vi "DumbDash Load Values.vi"(7 "Message Box":refnum<vi>, 10 "Robot":T1, 11 "Controls In":T2[](array[typedef])) -> ()   [LabVIEW 2017]
uses:
  DumbDash Control.ctl
  DumbDash Control Type.ctl
  Common Code/Robot Name.ctl
  <vilib>/Utility/sysdir.llb/System Directory Type.ctl
  <vilib>/Utility/config.llb/Read Key (Double).vi
  <vilib>/Utility/config.llb/Read Key (Boolean).vi
  <vilib>/Utility/config.llb/Read Key (String).vi
  <vilib>/Utility/config.llb/NI_LVConfig.lvlib
panel:
  out "file path":path
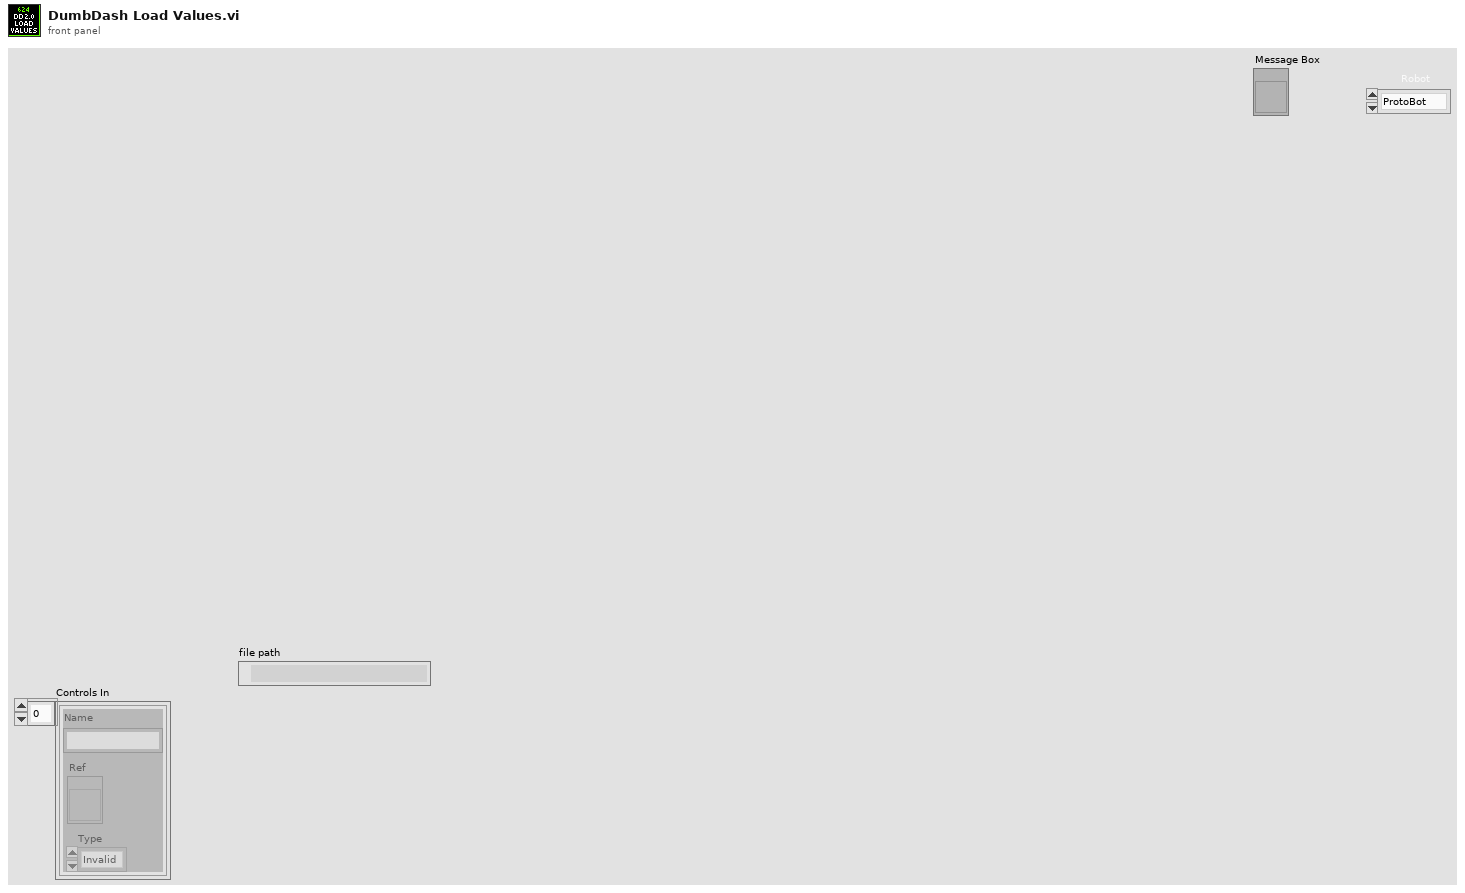
[diagram p1: front panel]
types:
  T1 = typedef "Robot Name.ctl" = enum16{"ProtoBot", "Main Robot", "Practice Robot"}
  T2 = typedef "DumbDash Control.ctl" = cluster{"Name":string, "Ref":refnum<vi>, "Type":T3}
  T3 = typedef "DumbDash Control Type.ctl" = enum16{"Invalid", "Number", "Boolean", "String"}
  T4 = typedef "System Directory Type.ctl" = i32
  T5 = typedef "NI_LVConfig.lvlib/Config Data RefNum.ctl" = refnum<k1>
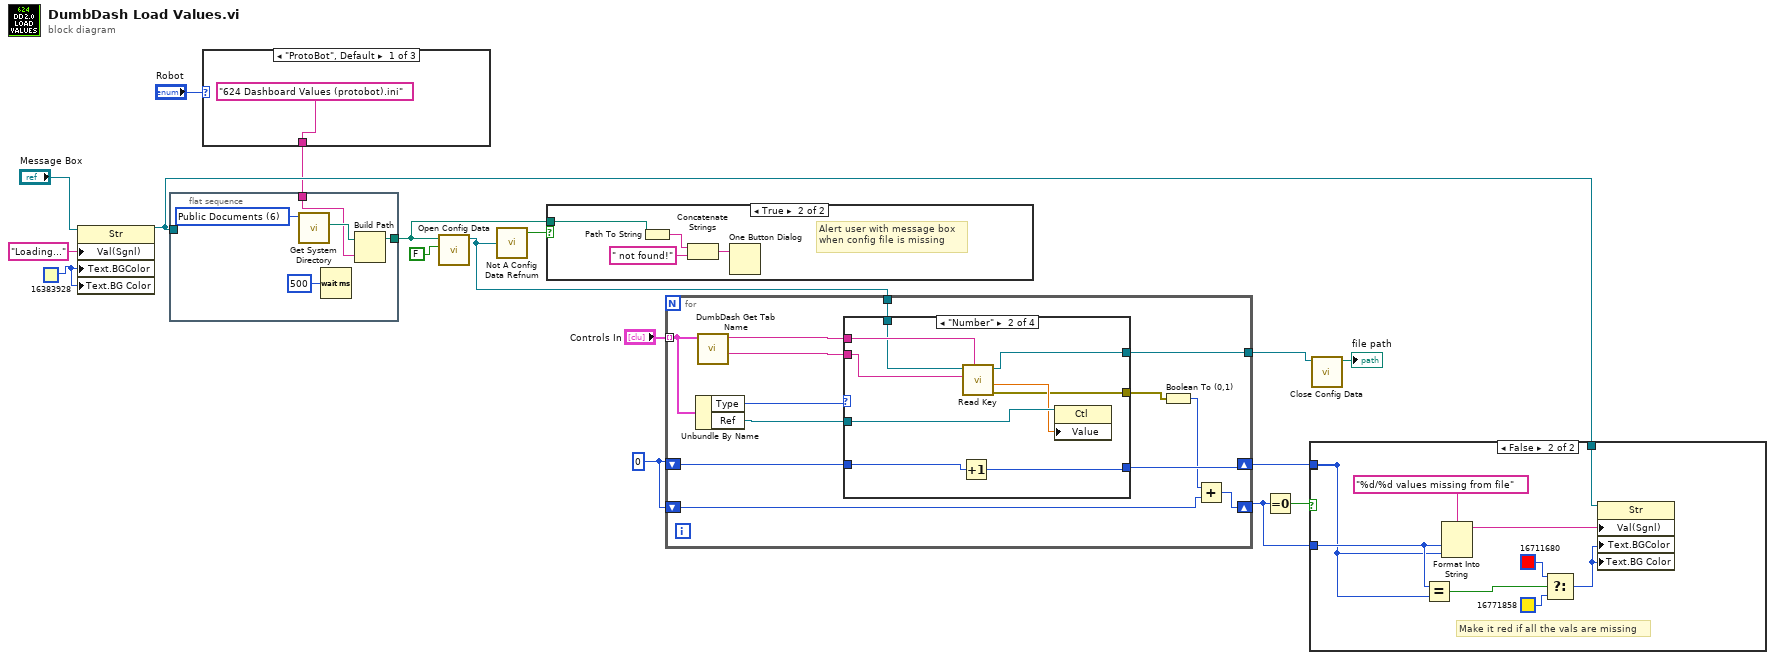
[diagram p0: block diagram]
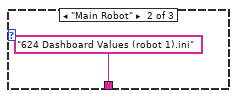
[diagram p2: hidden frame]
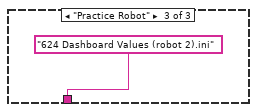
[diagram p3: hidden frame]
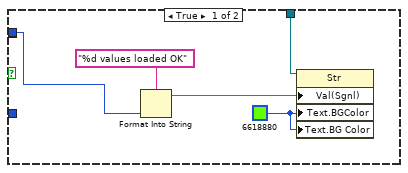
[diagram p5: hidden frame]
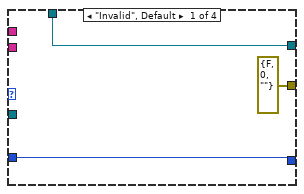
[diagram p6: hidden frame]
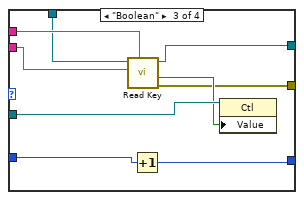
[diagram p7: hidden frame]
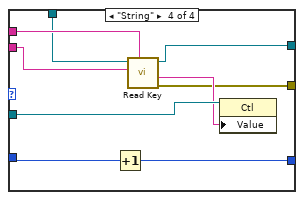
[diagram p8: hidden frame]
diagram:
  w10 = 0
  w11 = u32 16383928
  n1 = property class="Str"(reference="Message Box", "Val(Sgnl)"="Loading..." ("Text.Text"), "Text.BGColor"=w11, "Text.BG Color"=w11) -> (reference out=w6:refnum<vi>)  [unwired: 1 in, 1 out]
  n2 = flat-sequence {
    tunnel: [w20] -> w3
    tunnel: w6 -> [_]
    tunnel: w1 -> [w18]
    frame #0 {
      w22 = T4 6 items=["User Home"=0, "User Desktop"=1, "User Documents"=2, "User Application Data"=3, "User Preferences"=4, "User Temporary"=5, "Public Documents"=6, "Public Application Data"=7, "Public Preferences"=8, "Public Cache"=13, "System Core Libraries"=9, "System Installed Libraries"=10, "Application Files"=11, "Boot Volume Root"=12] ("system directory type")
      n3 = call <vilib>:"Get System Directory.vi"("system directory type"=w22) -> ("system directory"=w21:path)  [unwired: 10 in]
      n4 = Wait (ms)(milliseconds to wait=u32 500) -> ()  [unwired: 1 out]
      n5 = Build Path(base path=w21, name or relative path=w18) -> (appended path=w20:path)
    }
  }
  n6 = case shown="\"ProtoBot\", Default" "Robot" {
    tunnel: ["624 Dashboard Values (protobot).ini" ("name or relative path") "624 Dashboard Values (robot 1).ini" ("name or relative path") "624 Dashboard Values (robot 2).ini" ("name or relative path")] -> w1
    frame "ProtoBot", Default {
    }
    frame "Main Robot" {
    }
    frame "Practice Robot" {
    }
  }
  n7 = call <vilib>:"Open Config Data.vi"("create file if necessary (T)"=FALSE, "configuration file path"=w3) -> ("refnum"=w5:T5)  [unwired: 7 in, 2 out]
  n8 = call <vilib>:"Not A Config Data Refnum.vi"("refnum"=w5) -> ("not a config data refnum"=w4:bool)
  n9 = case shown="True" w4 {
    tunnel: w3 -> [_ w26]
    frame False {
    }
    frame True {
      # "Alert user with message box\nwhen config file is missing"
      n10 = Path To String(path=w26) -> (string=w29:string)
      n11 = Concatenate Strings(w29, " not found!" ("string")) -> (w27:string)
      n12 = One Button Dialog(message=w27) -> ()  [unwired: 1 in, 1 out]
    }
  }
  n13 = for {
    tunnel: "Controls In" -> [w38] mode=indexing
    tunnel: w5 -> [w41]
    tunnel: [w37] -> w16
    shift-right: [w34] -> w8
    shift-left: w10 -> [w35]
    shift-right: [w30] -> w7
    shift-left: w10 -> [w31]
    n14 = Unbundle By Name(w38) -> ("Type"=w39:T3, "Ref"=w36:refnum<vi>)
    n15 = call "DumbDash Get Tab Name.vi"("Cluster"=w38) -> ("Rest of Name"=w40:string, "Tab Name"=w42:string)  [unwired: 9 in]
    n16 = case shown="\"Number\"" w39 {
      tunnel: w42 -> [_ w54 w63 w72]
      tunnel: w41 -> [w45 w53 w62 w71]
      tunnel: w40 -> [_ w52 w61 w70]
      tunnel: [w45 w51 w60 w69] -> w37
      tunnel: w36 -> [_ w50 w59 w68]
      tunnel: w35 -> [w44 w48 w57 w66]
      tunnel: [w44 w47 w56 w65] -> w34
      tunnel: [errorcluster {"status"=FALSE, "code"=0, "source"=""} ("error out") w46 w55 w64] -> w33
      frame "Invalid", Default {
      }
      frame "Number" {
        n17 = Increment(x=w48) -> (x+1=w47:i32)
        n18 = call-poly <vilib>:"Read Key.vi"("section"=w54, "key"=w52, "refnum"=w53) -> ("error out"=w46:errorcluster, "value"=w49:dbl, "refnum out"=w51:T5)  [unwired: 5 in, 1 out]
        n19 = property class="Ctl"(reference=w50, "Value"=w49) -> ()  [unwired: 1 in, 2 out]
      }
      frame "Boolean" {
        n20 = call-poly <vilib>:"Read Key.vi"("section"=w63, "key"=w61, "refnum"=w62) -> ("error out"=w55:errorcluster, "value"=w58:bool, "refnum out"=w60:T5)  [unwired: 5 in, 1 out]
        n21 = Increment(x=w57) -> (x+1=w56:i32)
        n22 = property class="Ctl"(reference=w59, "Value"=w58) -> ()  [unwired: 1 in, 2 out]
      }
      frame "String" {
        n23 = Increment(x=w66) -> (x+1=w65:i32)
        n24 = call-poly <vilib>:"Read Key.vi"("section"=w72, "key"=w70, "refnum"=w71) -> ("error out"=w64:errorcluster, "value"=w67:string, "refnum out"=w69:T5)  [unwired: 5 in, 1 out]
        n25 = property class="Ctl"(reference=w68, "Value"=w67) -> ()  [unwired: 1 in, 2 out]
      }
    }
    n26 = Boolean To (0,1)(Boolean=w33) -> (0, 1=w32:i16)
    n27 = Add(x=w32, y=w31) -> (x+y=w30:i32)
  }
  n28 = Equal To 0?(x=w7) -> (x = 0?=w9:bool)
  n29 = case shown="False" w9 {
    tunnel: [w74 w82] -> _
    tunnel: w8 -> [w74 w82]
    tunnel: w7 -> [_ w83]
    tunnel: w6 -> [w73 w84]
    frame True {
      w75 = u32 6618880
      n30 = Format Into String(format string="%d values loaded OK", w74) -> (resulting string=w76:string)  [unwired: 2 in, 1 out]
      n31 = property class="Str"(reference=w73, "Val(Sgnl)"=w76, "Text.BGColor"=w75, "Text.BG Color"=w75) -> ()  [unwired: 1 in, 2 out]
    }
    frame False {
      # "Make it red if all the vals are missing"
      n32 = Equal?(x=w83, y=w82) -> (x = y?=w81:bool)
      n33 = Format Into String(format string="%d/%d values missing from file", w83, w82) -> (resulting string=w85:string)  [unwired: 2 in, 1 out]
      n34 = Select(t=u32 16711680, s=w81, f=u32 16771858) -> (s? t:f=w78:u32)
      n35 = property class="Str"(reference=w84, "Val(Sgnl)"=w85, "Text.BGColor"=w78, "Text.BG Color"=w78) -> ()  [unwired: 1 in, 2 out]
    }
  }
  n36 = call <vilib>:"Close Config Data.vi"("refnum"=w16) -> ("file path"=→"file path":path)  [unwired: 9 in, 1 out]
